vi "MS_on_off_sorting_power.vi"(0 "IR_off_q_in":refnum<queue>, 1 "IR_off_q_error_in":errorcluster, 2 "IR_on_q_in":refnum<queue>, 3 "IR_on_q_error_in":errorcluster, 4 "Power_q_in":refnum<queue>, 5 "Power_q_error_in":errorcluster, 6 "Number of sweeps":i32, 10 "Waveform + Power":cluster{"Waveform Graph":waveform(dbl), dbl}) -> (14 "IR_off_q_out":refnum<queue>, 15 "IR_off_q_error_out":errorcluster, 16 "IR_on_q_out":refnum<queue>, 17 "IR_on_q_error_out":errorcluster, 18 "Power_q_out":refnum<queue>, 19 "Power_q_error_out":errorcluster)   [LabVIEW 2020]
panel:
  out "Numeric":dbl
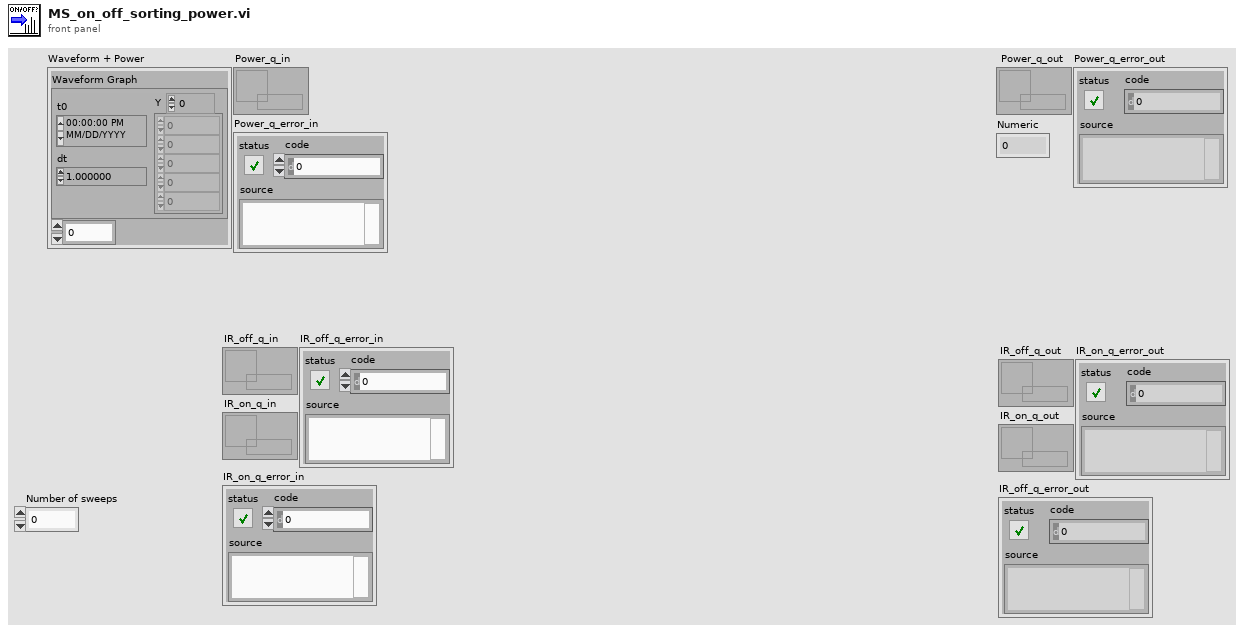
[diagram p1: front panel]
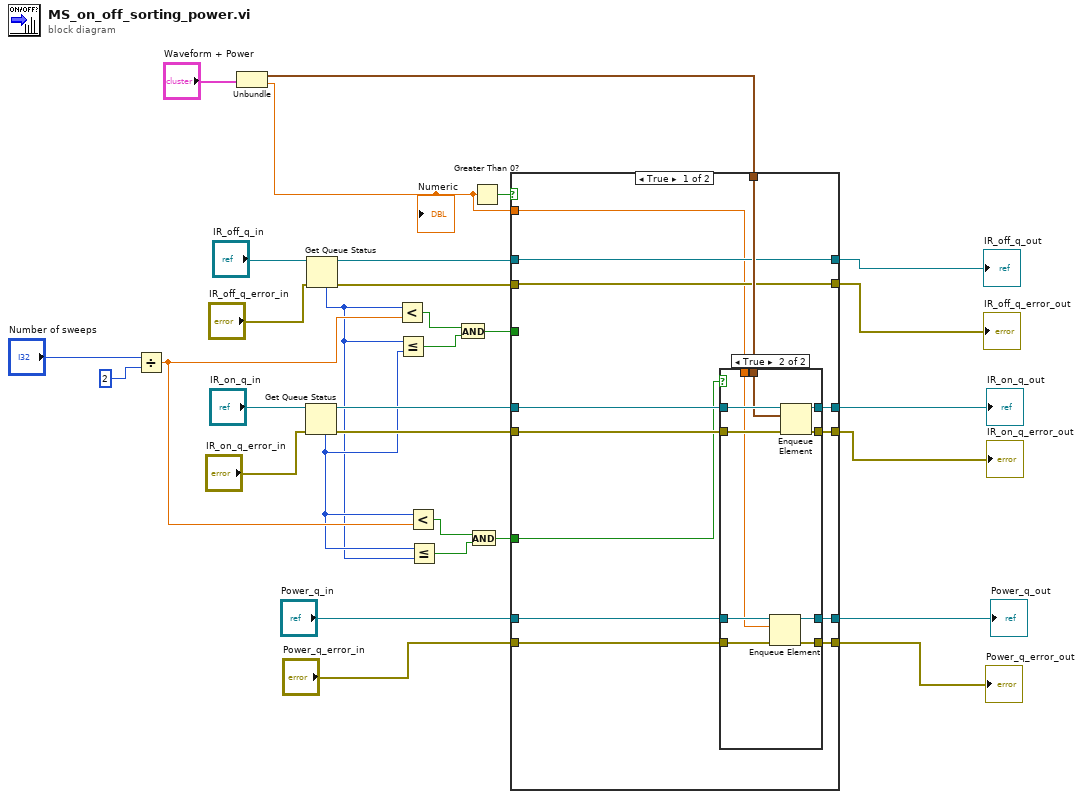
[diagram p0: block diagram]
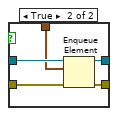
[diagram p4: hidden frame]
diagram:
  n1 = Divide(x="Number of sweeps", y=2) -> (x/y=w9:dbl)
  n2 = Unbundle("Waveform + Power") -> ("Waveform Graph"=w29:waveform(dbl), w3:dbl)
  "Numeric" <- w3
  n3 = Get Queue Status(queue="IR_on_q_in", error in (no error)="IR_on_q_error_in") -> (queue out=w20:refnum<queue>, error out=w19:errorcluster, # elements in queue=w8:i32)  [unwired: 1 in, 5 out]
  n4 = Get Queue Status(queue="IR_off_q_in", error in (no error)="IR_off_q_error_in") -> (queue out=w23:refnum<queue>, error out=w24:errorcluster, # elements in queue=w7:i32)  [unwired: 1 in, 5 out]
  n5 = Less?(x=w7, y=w9) -> (x < y?=w11:bool)
  n6 = Less Or Equal?(x=w7, y=w8) -> (x <= y?=w10:bool)
  n7 = Less?(x=w8, y=w9) -> (x < y?=w14:bool)
  n8 = Less Or Equal?(x=w8, y=w7) -> (x <= y?=w13:bool)
  n9 = And(x=w11, y=w10) -> (x .and. y?=w6:bool)
  n10 = And(x=w14, y=w13) -> (x .and. y?=w12:bool)
  n11 = Greater Than 0?(x=w3) -> (x > 0?=w31:bool)
  n12 = case shown="True" w31 {
    tunnel: w23 -> [w39 w68]
    tunnel: w24 -> [w38 w67]
    tunnel: w20 -> [w44 w63]
    tunnel: w19 -> [w42 w62]
    tunnel: [w39 w66] -> w28
    tunnel: [w38 w65] -> w27
    tunnel: w29 -> [w40 w64]
    tunnel: [w43 w63] -> w26
    tunnel: [w41 w62] -> w25
    tunnel: w12 -> [w37 _]
    tunnel: w6 -> [_ w61]
    tunnel: "Power_q_in" -> [w36 w60]
    tunnel: "Power_q_error_in" -> [w35 w59]
    tunnel: [w34 w60] -> w2
    tunnel: [w33 w59] -> w1
    tunnel: w3 -> [w32 _]
    frame True {
      n13 = case shown="True" w37 {
        tunnel: w44 -> [w48 w58]
        tunnel: [w48 w57] -> w43
        tunnel: w42 -> [w47 w56]
        tunnel: [w47 w55] -> w41
        tunnel: w40 -> [_ w54]
        tunnel: w36 -> [w46 w53]
        tunnel: w35 -> [w45 w52]
        tunnel: [w46 w51] -> w34
        tunnel: [w45 w50] -> w33
        tunnel: w32 -> [_ w49]
        frame False {
        }
        frame True {
          n14 = Enqueue Element(queue=w53, element=w49, error in (no error)=w52) -> (queue out=w51:refnum<queue>, error out=w50:errorcluster)  [unwired: 1 in, 1 out]
          n15 = Enqueue Element(queue=w58, element=w54, error in (no error)=w56) -> (queue out=w57:refnum<queue>, error out=w55:errorcluster)  [unwired: 1 in, 1 out]
        }
      }
    }
    frame False {
      n16 = case shown="False" w61 {
        tunnel: w68 -> [w70 w75]
        tunnel: w67 -> [w69 w74]
        tunnel: [w70 w73] -> w66
        tunnel: [w69 w72] -> w65
        tunnel: w64 -> [_ w71]
        frame False {
        }
        frame True {
          n17 = Enqueue Element(queue=w75, element=w71, error in (no error)=w74) -> (queue out=w73:refnum<queue>, error out=w72:errorcluster)  [unwired: 1 in, 1 out]
        }
      }
    }
  }
  "IR_off_q_out" <- w28
  "IR_on_q_out" <- w26
  "IR_on_q_error_out" <- w25
  "IR_off_q_error_out" <- w27
  "Power_q_out" <- w2
  "Power_q_error_out" <- w1
